vi "Configure VIPB Build.vi"(8 "error in (no error)":errorcluster, 10 "JSON string":string) -> (0 "error out":errorcluster, 3 "VIPB Build out":refnum<class "VIPB Build.lvclass">)   [LabVIEW 2014, in "VIPB Build.lvclass"]
uses:
  VIPB Build.lvclass
  Shared/Controls/VIPB Build - STYP.ctl
  VIPB Build.lvclass/VIPB Build.ctl
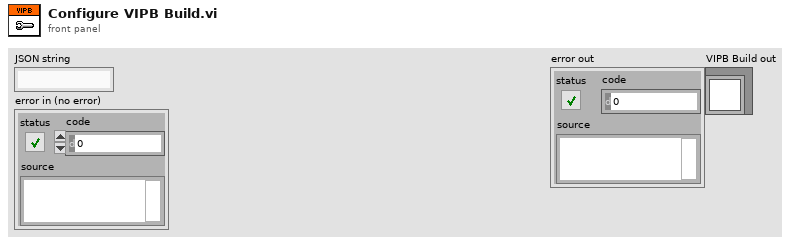
[diagram p1: front panel]
types:
  T1 = typedef "VIPB Build - STYP.ctl" = cluster{"VIPB Path":string, "Install after build":bool, "LabVIEW Version":string}
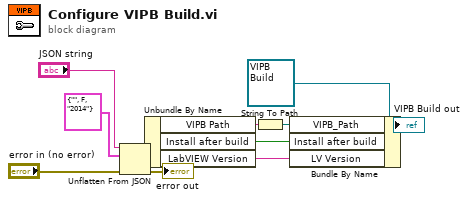
[diagram p0: block diagram]
diagram:
  n1 = Unflatten From JSON(JSON string="JSON string", type and defaults=T1 {"VIPB Path"="", "Install after build"=FALSE, "LabVIEW Version"="2014"} ("VIPB Build"), error in (no error)="error in (no error)") -> (value=w7:T1, error out=→"error out":errorcluster)  [unwired: 4 in]
  n2 = Unbundle By Name(w7) -> ("VIPB Path"=w5:string, "Install after build"=w2:bool, "LabVIEW Version"=w1:string)
  n3 = String To Path(string=w5) -> (path=w4:path)
  n4 = Bundle By Name(cluster=refnum<class "VIPB Build.lvclass"> refnum ("VIPB Build out"), "VIPB_Path"=w4, "Install after build"=w2, "LV Version"=w1) -> (→"VIPB Build out":refnum<class "VIPB Build.lvclass">)
